vi "experimental header read tester.vi"() -> ()   [LabVIEW 2017]
uses:
  User Interface/Visualisation/Functional Imaging Viewer/SubVIs/Experiment header interface/Typedefs/Header parameters cluster-ALL.ctl
  User Interface/Visualisation/Functional Imaging Viewer/SubVIs/Experiment header interface/Typedefs/Header subclusters/Header params -Login.ctl
  User Interface/Visualisation/Functional Imaging Viewer/SubVIs/Experiment header interface/Typedefs/Header subclusters/Header params-Global Parameters.ctl
  User Interface/Misc/Experiment Type.ctl
  User Interface/Visualisation/Functional Imaging Viewer/SubVIs/Experiment header interface/Typedefs/Header subclusters/Header params-Imaging Modes.ctl
  User Interface/Visualisation/Functional Imaging Viewer/SubVIs/Experiment header interface/Typedefs/Header subclusters/Header params-Time Series.ctl
  User Interface/Visualisation/Functional Imaging Viewer/SubVIs/Experiment header interface/Typedefs/Header subclusters/Header params-Basic image meta data.ctl
  Typedefs/Frame Size.ctl
  User Interface/Visualisation/Functional Imaging Viewer/SubVIs/Experiment header interface/Typedefs/Header subclusters/Header params-Motor Z-stack.ctl
  User Interface/Visualisation/Functional Imaging Viewer/SubVIs/Experiment header interface/Typedefs/Header subclusters/Header params-AOL Z-stack.ctl
  User Interface/Visualisation/Functional Imaging Viewer/SubVIs/Experiment header interface/Typedefs/Header subclusters/Header params-Functional Imaging.ctl
  Typedefs/Functional Mode.ctl
  Typedefs/AOL modes.ctl
  Typedefs/Plane Mode.ctl
  User Interface/Visualisation/Functional Imaging Viewer/SubVIs/Experiment header interface/Typedefs/Header subclusters/Header params-Calibration Setup.ctl
  User Interface/Visualisation/Functional Imaging Viewer/SubVIs/Experiment header interface/Typedefs/Header subclusters/Header params-statistics.ctl
  User Interface/Misc/Biology Information.ctl
  User Interface/Visualisation/Functional Imaging Viewer/SubVIs/Experiment header interface/Typedefs/Header file section refs.ctl
  User Interface/Visualisation/Functional Imaging Viewer/SubVIs/Experiment header interface/Typedefs/Header file sections.ctl
  User Interface/Visualisation/Functional Imaging Viewer/SubVIs/Experiment header interface/Typedefs/Header file actions.ctl
panel:
  in  "Experiment data folder path":path
  out "Section Refs":T1[](array[typedef])
  out "All header parameters in":T2 {"VOLUME IMAGING"."Plane Mode" items=["XY Plane", "XZ Plane", "YZ Plane", "arbitraryplane"]; "VOLUME IMAGING"."Basic Image meta data"."Frame Size" items=["100X100"=100, "128X128"=128, "200X200"=200, "256X256"=256, "512X512"=512, "1024x1024"=1024, "2048x2048"=2048]; "AOL Z-STACK"."Hdr Basic Image meta data"."Frame Size" items=["100X100"=100, "128X128"=128, "200X200"=200, "256X256"=256, "512X512"=512, "1024x1024"=1024, "2048x2048"=2048]; "MOTOR Z-STACK"."Hdr Basic Image meta data"."Frame Size" items=["100X100"=100, "128X128"=128, "200X200"=200, "256X256"=256, "512X512"=512, "1024x1024"=1024, "2048x2048"=2048]; "FUNCTIONAL IMAGING"."Plane Mode" items=["XY Plane", "XZ Plane", "YZ Plane", "arbitraryplane"]; "FUNCTIONAL IMAGING"."Basic Image meta data"."Frame Size" items=["100X100"=100, "128X128"=128, "200X200"=200, "256X256"=256, "512X512"=512, "1024x1024"=1024, "2048x2048"=2048]; "TIME SERIES"."Basic Image meta data"."Frame Size" items=["100X100"=100, "128X128"=128, "200X200"=200, "256X256"=256, "512X512"=512, "1024x1024"=1024, "2048x2048"=2048]}
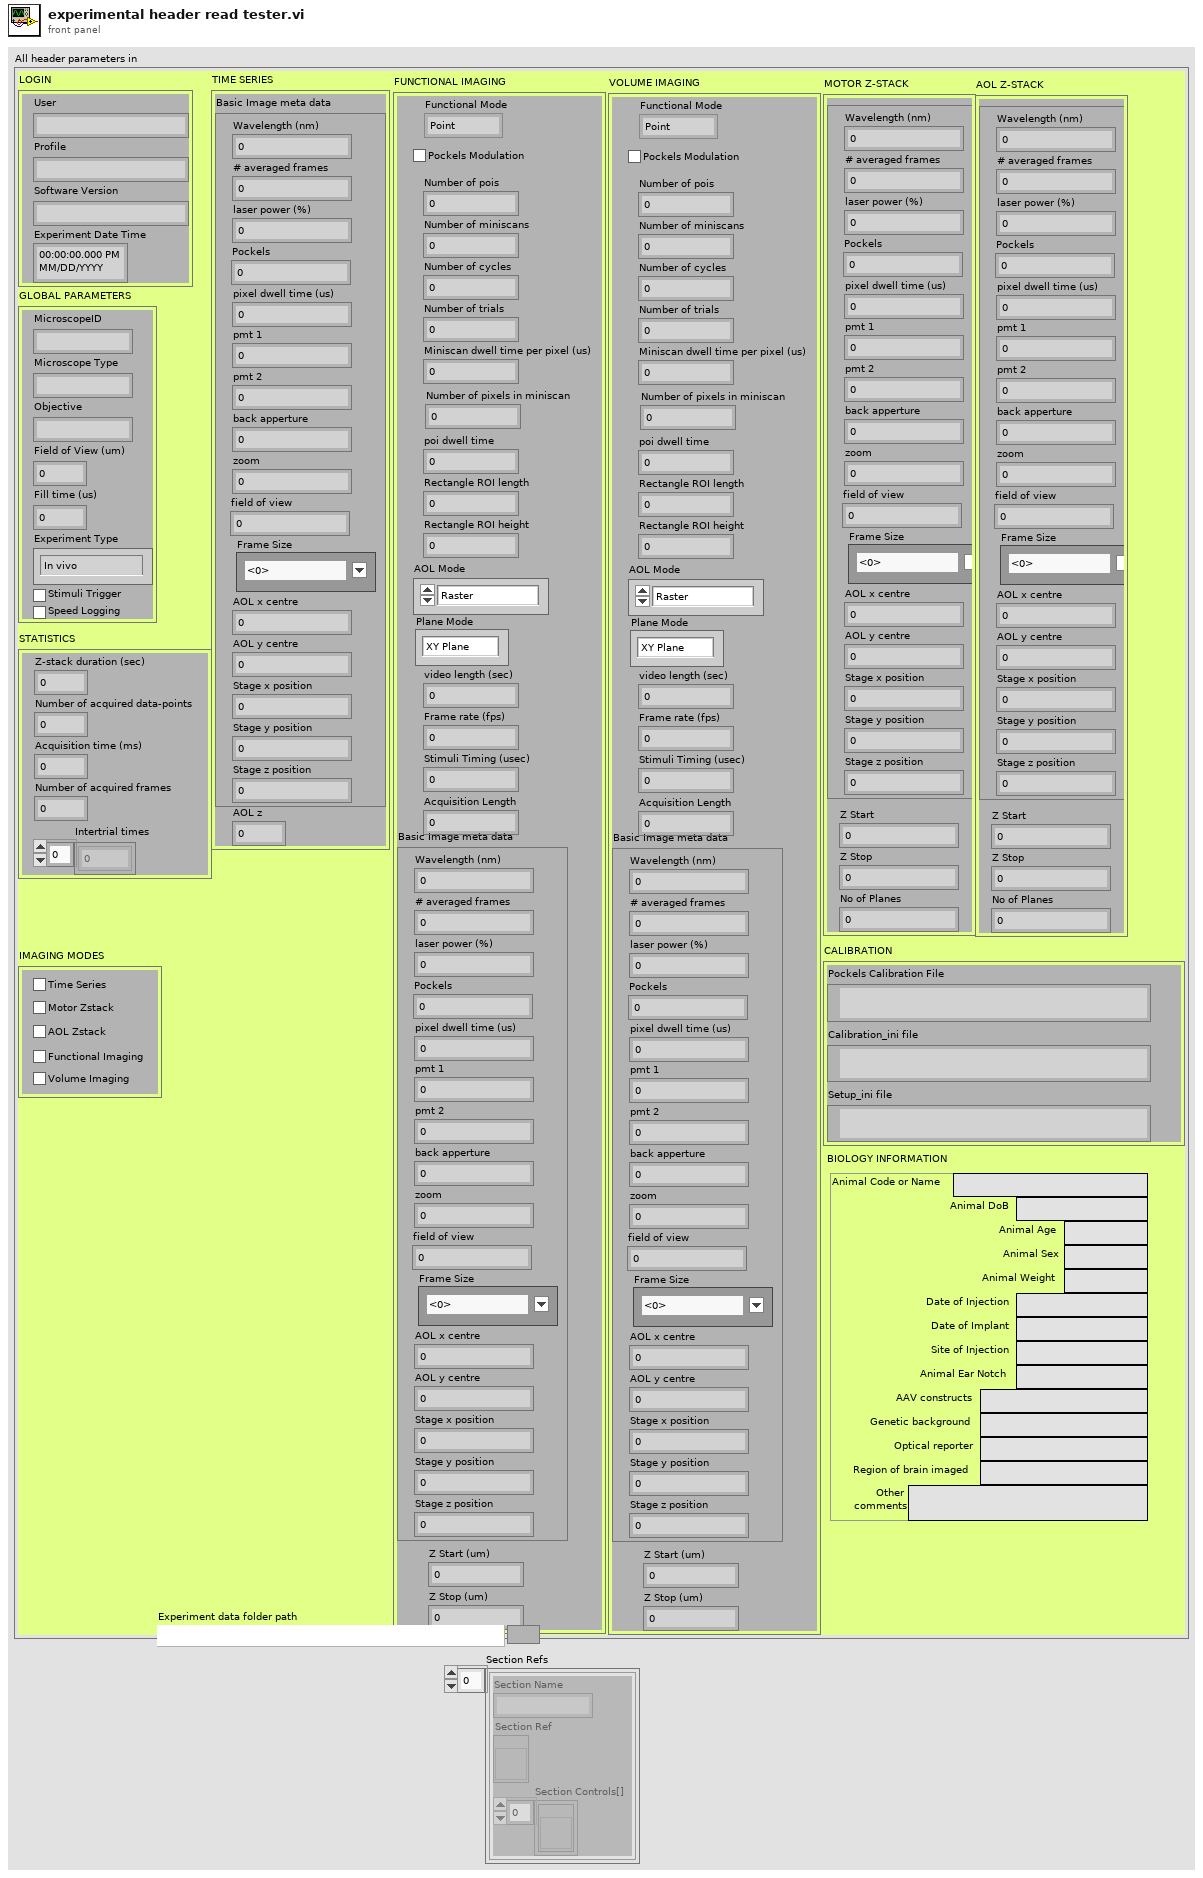
[diagram p1: front panel]
types:
  T1 = typedef "Header file section refs.ctl" = cluster{"Section Name":string, "Section Ref":refnum<vi>, "Section Controls[]":refnum<vi>[]}
  T2 = typedef "Header parameters cluster-ALL.ctl" = cluster{"LOGIN":T3, "GLOBAL PARAMETERS":T4, "IMAGING MODES":T6, "TIME SERIES":T7, "MOTOR Z-STACK ":T10, "AOL Z-STACK":T11, "FUNCTIONAL IMAGING":T12, "VOLUME IMAGING":T12, "CALIBRATION":T16, "STATISTICS":T17, "BIOLOGY INFORMATION":T18}
  T3 = typedef "Header params -Login.ctl" = cluster{"User":string, "Profile":string, "Software Version":string, "Experiment Date Time":timestamp}
  T4 = typedef "Header params-Global Parameters.ctl" = cluster{"MicroscopeID":string, "Microscope Type":string, "Objective":string, "Field of View (um)":dbl, "Fill time (us)":dbl, "Experiment Type":T5, "Stimuli Trigger":bool, "Speed Logging":bool}
  T5 = typedef "Experiment Type.ctl" = enum16{"In vivo", "In vitro", "Testing", "Calibration", "Other"}
  T6 = typedef "Header params-Imaging Modes.ctl" = cluster{"Time Series":bool, "Motor Zstack":bool, "AOL Zstack":bool, "Functional Imaging":bool, "Volume Imaging":bool}
  T7 = typedef "Header params-Time Series.ctl" = cluster{"Basic Image meta data":T8, "AOL z":dbl}
  T8 = typedef "Header params-Basic image meta data.ctl" = cluster{"Wavelength (nm)":dbl, "# averaged frames":dbl, "laser power (%)":dbl, "Pockels":dbl, "pixel dwell time (us)":dbl, "pmt 1":dbl, "pmt 2":dbl, "back apperture":dbl, "zoom":dbl, "field of view":dbl, "Frame Size":T9, "AOL x centre":dbl, "AOL y centre":dbl, "Stage x position":dbl, "Stage y position":dbl, "Stage z position":dbl}
  T9 = typedef "Frame Size.ctl" = u16
  T10 = typedef "Header params-Motor Z-stack.ctl" = cluster{"Hdr Basic Image meta data":T8, "Z Start":dbl, "Z Stop":dbl, "No of Planes":i32}
  T11 = typedef "Header params-AOL Z-stack.ctl" = cluster{"Hdr Basic Image meta data":T8, "Z Start":dbl, "Z Stop":dbl, "No of Planes":i32}
  T12 = typedef "Header params-Functional Imaging.ctl" = cluster{"Functional Mode":T13, "Pockels Modulation":bool, "Number of pois":dbl, "Number of miniscans":dbl, "Number of cycles":dbl, "Number of trials":dbl, "Miniscan dwell time per pixel (us)":dbl, "Number of pixels in miniscan":dbl, "poi dwell time":dbl, "Rectangle ROI length":dbl, "Rectangle ROI height":dbl, "AOL Mode":T14, "Plane Mode":T15, "video length (sec)":dbl, "Frame rate (fps)":dbl, "Stimuli Timing (usec)":dbl, "Acquisition Length":dbl, "Basic Image meta data":T8, "Z Start (um)":dbl, "Z Stop (um)":dbl}
  T13 = typedef "Functional Mode.ctl" = enum16{"Point", "Line", "Patch", "Plane", "Volume"}
  T14 = typedef "AOL modes.ctl" = enum16{"Raster", "Structural", "Pointing", "Mini Scan", "Alignment"}
  T15 = typedef "Plane Mode.ctl" = u16
  T16 = typedef "Header params-Calibration Setup.ctl" = cluster{"Pockels Calibration File":path, "Calibration_ini file":path, "Setup_ini file":path}
  T17 = typedef "Header params-statistics.ctl" = cluster{"Z-stack duration (sec)":dbl, "Number of acquired data-points":dbl, "Acquisition time (ms)":dbl, "Number of acquired frames":dbl, "Intertrial times":dbl[]}
  T18 = typedef "Biology Information.ctl" = cluster{"Animal Code or Name":string, "Animal DoB":string, "Animal Age":string, "Animal Sex":string, "Animal Weight":string, "Date of Injection":string, "Date of Implant":string, "Site of Injection":string, "Animal Ear Notch":string, "AAV constructs":string, "Genetic background":string, "Optical reporter":string, "Region of brain imaged":string, "Other \ncomments":string}
  T19 = typedef "Header file actions.ctl" = enum16{"Create", "Open", "Read All", "Read Section", "Write All", "Write Section", "Close"}
  T20 = typedef "Header file sections.ctl" = enum16{"ALL SECTIONS", "LOGIN", "GLOBAL PARAMETERS", "IMAGING MODES", "TIME SERIES", "MOTOR Z-STACK", "AOL Z-STACK", "FUNCTIONAL IMAGING", "VOLUME IMAGING", "CALIBRATION", "STATISTICS", "BIOLOGY INFORMATION"}
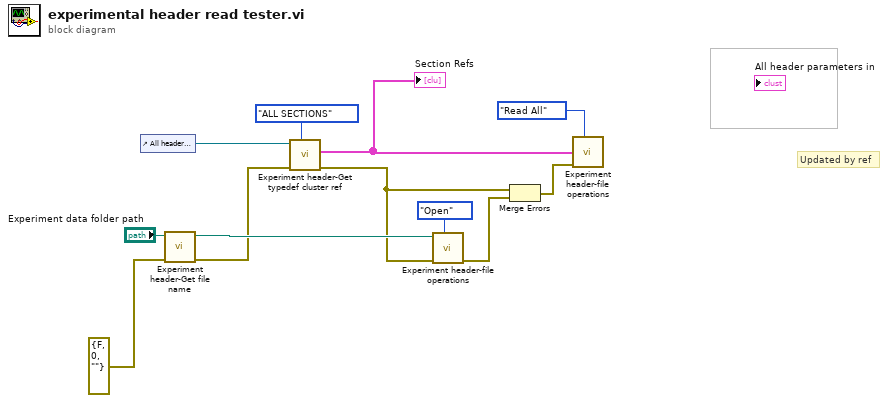
[diagram p0: block diagram]
diagram:
  # "Updated by ref"
  n1 = control-ref of="All header parameters in"() -> (w9:refnum<vi>)
  n2 = call "Experiment header-Get file name.vi"("error in (no error)"=errorcluster {"status"=FALSE, "code"=0, "source"=""}, "Experiment data folder path"="Experiment data folder path") -> ("error out"=w7:errorcluster, "Header File Path"=w10:path)  [unwired: 8 in]
  n3 = call "Experiment header-Get typedef cluster ref.vi"("Header file sections"=Header_file_sections."ALL SECTIONS", "error in (no error)"=w7, "All header parameters / Header module interface cluster"=w9) -> ("error out"=w3:errorcluster, "Section Refs"=w2:T1[])  [unwired: 5 in, 2 out]
  "Section Refs" <- w2
  n4 = call "Experiment header-file operations.vi"("Header file actions"=Header_file_actions."Open", "error in (no error)"=w3, "Path"=w10) -> ("error out"=w6:errorcluster)  [unwired: 8 in]
  n5 = Merge Errors(w3, w6) -> (w5:errorcluster)
  n6 = call "Experiment header-file operations.vi"("Header file actions"=Header_file_actions."Read All", "error in (no error)"=w5, "Section Refs"=w2) -> ()  [unwired: 8 in, 1 out]
